vi "Reassign Bounds.vi"(6 "Offset from New (100)":i16=100, 9 "New Top":i16, 10 "New Left":i16, 11 "Bounds in":T1) -> (3 "Bounds out":T1)   [LabVIEW 2020]
uses:
  <vilib>/Utility/miscctls.llb/LVRectTypeDef.ctl
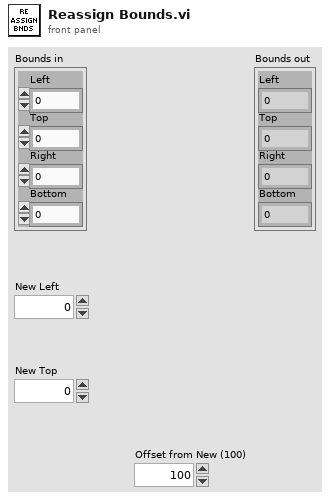
[diagram p1: front panel]
types:
  T1 = typedef "LVRectTypeDef.ctl" = cluster{"Left":i16, "Top":i16, "Right":i16, "Bottom":i16}
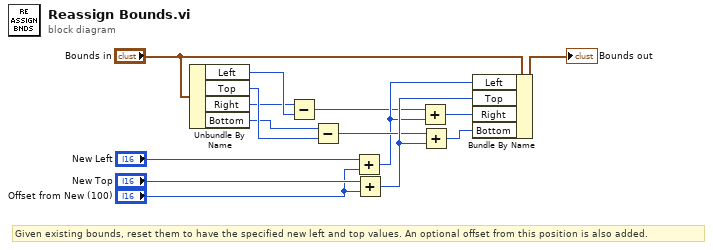
[diagram p0: block diagram]
diagram:
  # "Given existing bounds, reset them to have the specified new left and top values. An optional offset from this position is also added."
  n1 = Unbundle By Name("Bounds in") -> ("Left"=w2:i16, "Top"=w4:i16, "Right"=w1:i16, "Bottom"=w3:i16)
  n2 = Subtract(x=w1, y=w2) -> (x-y=w7:i16)
  n3 = Subtract(x=w3, y=w4) -> (x-y=w10:i16)
  n4 = Add(x="New Left", y="Offset from New (100)") -> (x+y=w8:i16)
  n5 = Add(x="New Top", y="Offset from New (100)") -> (x+y=w12:i16)
  n6 = Add(x=w7, y=w8) -> (x+y=w9:i16)
  n7 = Add(x=w10, y=w12) -> (x+y=w11:i16)
  n8 = Bundle By Name(cluster="Bounds in", "Left"=w8, "Top"=w12, "Right"=w9, "Bottom"=w11) -> (→"Bounds out":T1)
